vi "Get Error Handler.vi"(8 "error in (no error)":errorcluster, 11 "Process In":refnum<class "Helper Loop.lvclass">) -> (0 "error out":errorcluster, 2 "Error Handler":refnum<class "Error Handler Interface.lvclass">, 3 "Process Out":refnum<class "Helper Loop.lvclass">)   [LabVIEW 2020]
doc: "Returns the error handler configured for the process using the Set Error Handler.vi method."
uses:
  Helper Loop.lvclass
  Error Handler Interface/Error Handler Interface.lvclass
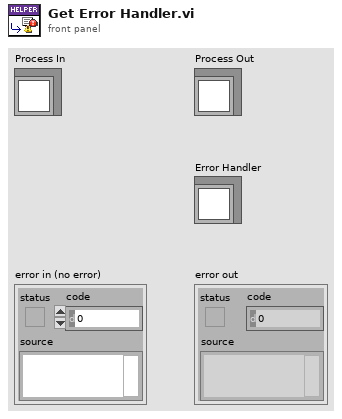
[diagram p1: front panel]
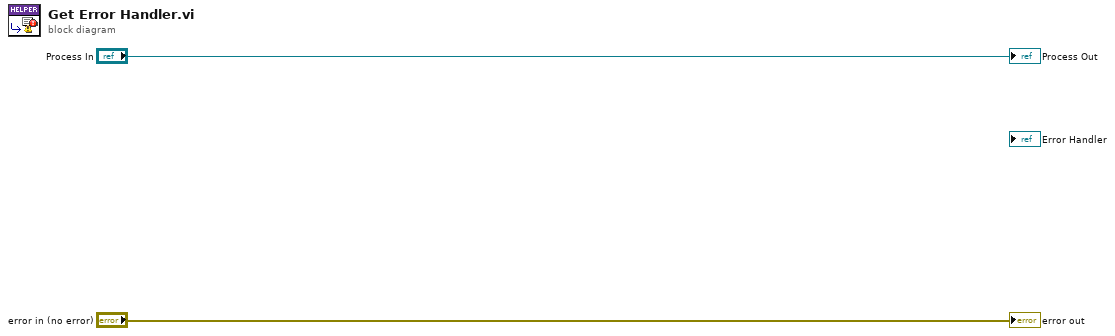
[diagram p0: block diagram]
diagram:
  "error out" <- "error in (no error)"
  "Process Out" <- "Process In"
